vi "TrajectoryConfig_AddConstraint.vi"(9 "Constraint":variant, 11 "inTRAJECTORY_CONFIG":T1 {"End Velocity" format="%20.4f"; "StartVelocity" format="%20.4f"; "Max Acceleration" format="%20.4f"; "MaxVelocity" format="%20.4f"}) -> (3 "outTRAJECTORY_CONFIG":T1 {"End Velocity" format="%20.4f"; "StartVelocity" format="%20.4f"; "Max Acceleration" format="%20.4f"; "MaxVelocity" format="%20.4f"})   [LabVIEW 2019, in "Trajectory_Library.lvlib"]
doc: "Add a constraint to this Trajectory Configuration\n\nParameters:\n - InTrajectoryConfig - The trajectory configuration data structure\n - Constraint -- Trajectory constraint converted to a variant\n\nReturns:\n - OutTrajectoryConfig - Modified trajectory configuration data structure"
uses:
  Trajectory_Library.lvlib
  TypeDef/TRAJ_CONFIG.ctl
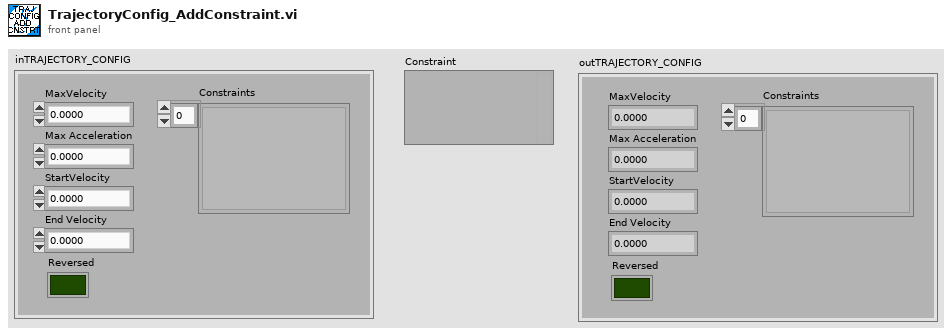
[diagram p1: front panel]
types:
  T1 = typedef "Trajectory_Library.lvlib/TRAJ_CONFIG.ctl" = cluster{"MaxVelocity":dbl, "Max Acceleration":dbl, "StartVelocity":dbl, "End Velocity":dbl, "Reversed":bool, "Constraints":variant[]}
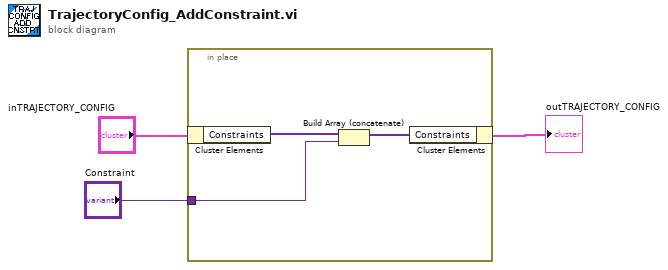
[diagram p0: block diagram]
diagram:
  n1 = in-place {
    in-place-border: "Constraint" -> [w4]
    n2 = in-place-cluster #1("inTRAJECTORY_CONFIG") -> ("Constraints"=w6:variant[])
    n3 = Build Array (concatenate)(w6, w4) -> (w5:variant[])
    n4 = in-place-cluster #1("Constraints"=w5) -> (→"outTRAJECTORY_CONFIG":T1)
  }
